vi "Save Text.vi"(8 "error in":errorcluster, 10 "text":string, 11 "JSON in":refnum<class "JSON.lvclass">) -> (0 "error out":errorcluster, 3 "JSON out":refnum<class "JSON.lvclass">)   [LabVIEW 2017, in "Report_lib.lvlib" / "JSON.lvclass"]
doc: "This method serves for \nwrite string into external\ntext file"
uses:
  JSON.lvclass
  JSON.lvclass/JSON.ctl
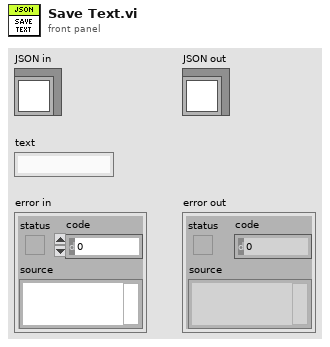
[diagram p1: front panel]
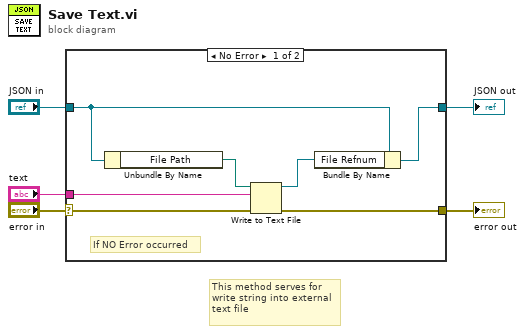
[diagram p0: block diagram]
diagram:
  # "This method serves for \nwrite string into external\ntext file"
  n1 = case shown="No Error" "error in" {
    selector: "error in" -> [w10 w14]
    tunnel: [w9 w14] -> w4
    tunnel: [w7 w13] -> w2
    tunnel: "JSON in" -> [w8 w13]
    tunnel: "text" -> [w11 _]
    frame No Error {
      # "If NO Error occurred"
      n2 = Unbundle By Name(w8) -> ("File Path"=w12:path)
      n3 = Write to Text File(file (use dialog)=w12, text=w11, error in=w10) -> (refnum out=w6:refnum<file>, error out=w9:errorcluster)  [unwired: 1 in, 1 out]
      n4 = Bundle By Name(cluster=w8, "File Refnum"=w6) -> (w7:refnum<class "JSON.lvclass">)
    }
    frame Error {
    }
  }
  "error out" <- w4
  "JSON out" <- w2
